vi "BRig_dataExp_Loop_T_ExpStruct.vi"() -> (2 "output_Loop_T_ExpStruct":i32)   [LabVIEW 2014]
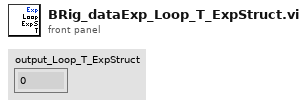
[diagram p1: front panel]
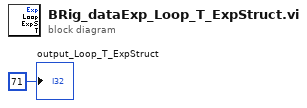
[diagram p0: block diagram]
diagram:
  "output_Loop_T_ExpStruct" <- 71 ("output_iBlock")
